vi "dbc-open-data-base.vi"(8 "error in (no error)":errorcluster, 9 "alias":string, 10 "dbc.path":path, 11 "dbc in":refnum<class "dbc.lvclass">) -> (0 "error out":errorcluster, 3 "dbc out":refnum<class "dbc.lvclass">)   [LabVIEW 2015, in "dbc.lvclass"]
uses:
  dbc.lvclass
  controls/dbc-file-data.ctl
  dbc.lvclass/dbc.ctl
  write-file-data.vi
  write-dbc-content.vi
  <vilib>/xnet/xnet.llb/XNET String To IO Name (Database Alias).vi
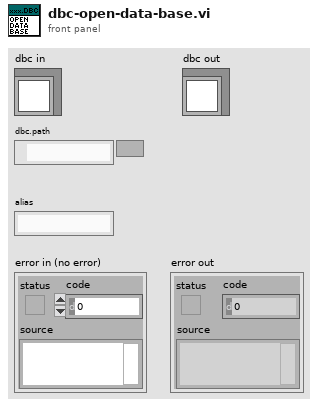
[diagram p1: front panel]
types:
  T1 = typedef "dbc-file-data.ctl" = cluster{"dbc.ref":refnum<k21>, "dbc.file":path, "alias":string}
  T2 = typedef "dbc-content-data.ctl" = cluster{"Number of Clusters":i32, "Number of Frames ":i32[], "Clusters":string[], "Frames":string[][], "Signals":string[][][], "Number of Signals":i32[][]}
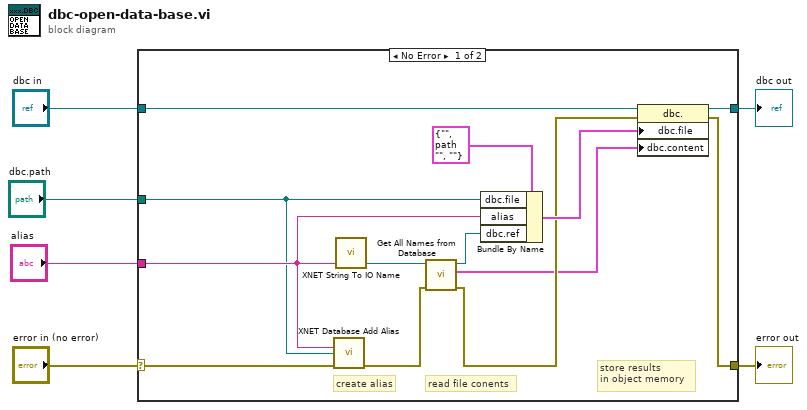
[diagram p0: block diagram]
diagram:
  n1 = case shown="No Error" "error in (no error)" {
    selector: "error in (no error)" -> [w16 w21]
    tunnel: [w12 w21] -> w5
    tunnel: [w18 w20] -> w3
    tunnel: "dbc in" -> [w19 w20]
    tunnel: "dbc.path" -> [w14 _]
    tunnel: "alias" -> [w15 _]
    frame No Error {
      # "store results\nin object memory"
      # "read file conents"
      # "create alias"
      n2 = call <vilib>:"XNET Database Add Alias.vi"("alias"=w15, "filepath"=w14, "error in (no error)"=w16) -> ("error out"=w9:errorcluster)  [unwired: 12 in]
      n3 = call-poly <vilib>:"XNET String To IO Name.vi"("string"=w15) -> ("XNET Database"=w13:refnum<k21>)  [unwired: 4 out]
      n4 = call "Get All Names from Database.vi"("error in (no error)"=w9, "database in (:memory:)"=w13) -> ("error out"=w8:errorcluster, "Cluster"=w7:T2, "XNET Database"=w10:refnum<k21>)  [unwired: 7 in]
      n5 = Bundle By Name(cluster=T1 {"dbc.ref"="", "dbc.file"=path "", "alias"=""} ("dbc.file"), "dbc.file"=w14, "alias"=w15, "dbc.ref"=w10) -> (w11:T1)
      n6 = property class="dbc."(reference=w19, error in=w8, "dbc.file"=w11, "dbc.content"=w7) -> (reference out=w18:refnum<class "dbc.lvclass">, error out=w12:errorcluster)
    }
    frame Error {
    }
  }
  "error out" <- w5
  "dbc out" <- w3
